vi "AlliGator Computer User-defined Quantity.vi"(6 "Init (F)":bool, 8 "Error In":errorcluster, 9 "Formula":string, 11 "Basic Quantities":sgl[](array[numeric])) -> (0 "Error Out":errorcluster, 3 "User-defined Quantity":sgl)   [LabVIEW 2021, in "AlliGator Phasor Plot.lvlib"]
doc: "Computes a user-defined quantity based on the basic quantities:\n\nf_!, f_2, a_1, a_2\ntau_phi, tau_m,\n<tau>_i, <tau>_a,\ntau_1, tau_@,\nT_laser, T_sync,\nN_gates,\ndt (gate separation)\nCh_INT (intensity of the INT channel)\nCh_G2 (intensity of the INT channel)"
uses:
  AlliGator Phasor Plot.lvlib
  <vilib>/gmath/NI_Gmath.lvlib
panel:
  # "see the AlliGator License on the block diagram (Ctrl+E or Window:Show Block Diagram)"
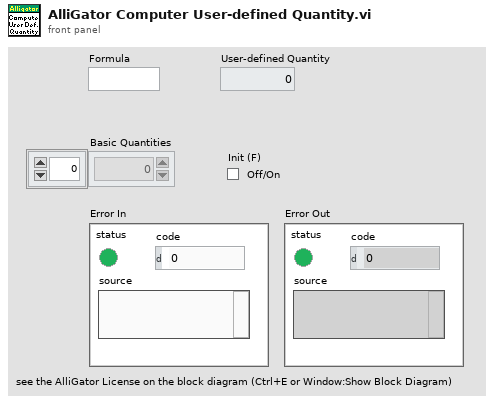
[diagram p1: front panel]
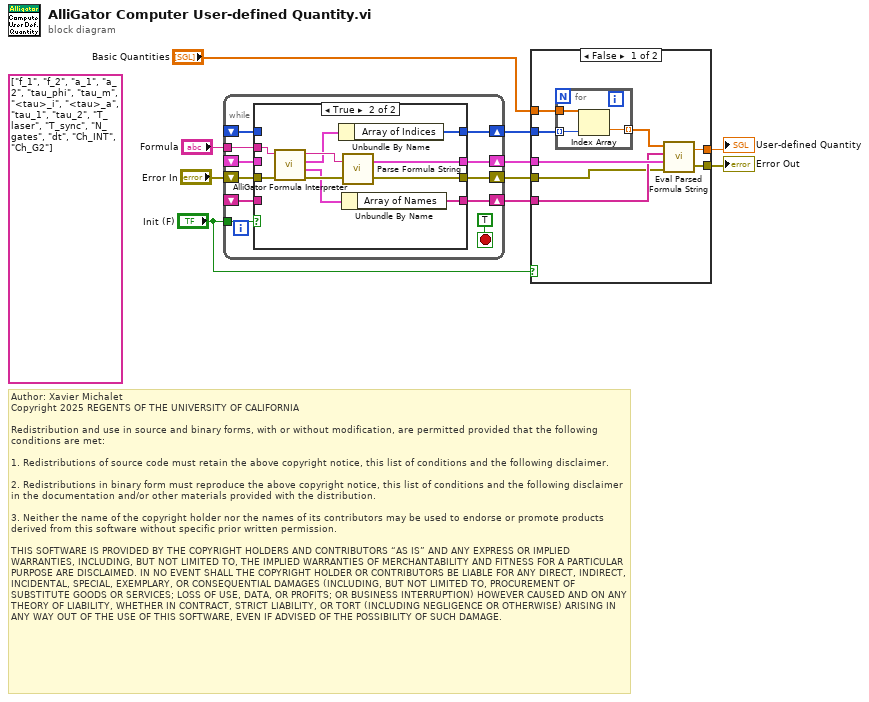
[diagram p0: block diagram]
diagram:
  (unwired) string[] ["f_1", "f_2", "a_1", "a_2", "tau_phi", "tau_m", "<tau>_i", "<tau>_a", "tau_1", "tau_2", "T_laser", "T_sync", "N_gates", "dt", "Ch_INT", "Ch_G2"] ("Basic Variable Names")
  # "Author: Xavier Michalet\nCopyright 2025 REGENTS OF THE UNIVERSITY OF CALIFORNIA\n\nRedistribution and use in source and binary forms, with or without modification, are permitted provided that the following conditions are met:\n\n1. Redistributions of source code must retain the above copyright notice, this list of conditions and the following disclaimer.\n\n2. Redistributions in binary form must reproduce the above copyright notice, this list of conditions and the following disclaimer in the documentation and/or other materials provided with the distribution.\n\n3. Neither the name of the copyright holder nor the names of its contributors may be used to endorse or promote products derived from this software without specific prior written permission.\n\nTHIS SOFTWARE IS PROVIDED BY THE COPYRIGHT HOLDERS AND CONTRIBUTORS “AS IS” AND ANY EXPRESS OR IMPLIED WARRANTIES, INCLUDING, BUT NOT LIMITED TO, THE IMPLIED WARRANTIES OF MERCHANTABILITY AND FITNESS FOR A PARTICULAR PURPOSE ARE DISCLAIMED. IN NO EVENT SHALL THE COPYRIGHT HOLDER OR CONTRIBUTORS BE LIABLE FOR ANY DIRECT, INDIRECT, INCIDENTAL, SPECIAL, EXEMPLARY, OR CONSEQUENTIAL DAMAGES (INCLUDING, BUT NOT LIMITED TO, PROCUREMENT OF SUBSTITUTE GOODS OR SERVICES; LOSS OF USE, DATA, OR PROFITS; OR BUSINESS INTERRUPTION) HOWEVER CAUSED AND ON ANY THEORY OF LIABILITY, WHETHER IN CONTRACT, STRICT LIABILITY, OR TORT (INCLUDING NEGLIGENCE OR OTHERWISE) ARISING IN ANY WAY OUT OF THE USE OF THIS SOFTWARE, EVEN IF ADVISED OF THE POSSIBILITY OF SUCH DAMAGE."
  n1 = while {
    tunnel: "Formula" -> [w21]
    shift-right: [w16] -> w4
    shift-left: "Error In" -> [w20]
    tunnel: "Init (F)" -> [w14]
    shift-right: [w19] -> w8
    shift-left: _ -> [w13]
    shift-right: [w18] -> w6
    shift-left: _ -> [w12]
    shift-right: [w17] -> w5
    shift-left: _ -> [w11]
    stop <- TRUE stop-if-true
    n2 = case shown="True" w14 {
      tunnel: w21 -> [_ w35]
      tunnel: w20 -> [w22 w34]
      tunnel: [w25 w30] -> w19
      tunnel: [w24 w29] -> w18
      tunnel: [w23 w27] -> w17
      tunnel: [w22 w26] -> w16
      tunnel: w13 -> [w25 _]
      tunnel: w12 -> [w24 _]
      tunnel: w11 -> [w23 _]
      frame False {
      }
      frame True {
        n3 = call "AlliGator Formula Interpreter.vi"("error in (no error)"=w34, "Original Formula"=w35) -> ("error out"=w32:errorcluster, "Variable Names"=w28:cluster{"Array of Names":string[]}, "Variable Indices"=w31:cluster{"Array of Indices":i32[]}, "Interpreted Formula"=w33:string)  [unwired: 5 in, 1 out]
        n4 = Unbundle By Name(w31) -> ("Array of Indices"=w30:i32[])
        n5 = Unbundle By Name(w28) -> ("Array of Names"=w27:string[])
        n6 = call <vilib>:"Parse Formula String.vi"("error in (no error)"=w32, "formula"=w33) -> ("error out"=w26:errorcluster, "Parsed Formula"=w29:cluster{"Table":i32[][], "Y Values":dbl[]})
      }
    }
  }
  n7 = case shown="False" "Init (F)" {
    tunnel: w8 -> [w42 _]
    tunnel: "Basic Quantities" -> [w41 _]
    tunnel: w6 -> [w40 _]
    tunnel: w5 -> [w39 _]
    tunnel: w4 -> [w38 w47]
    tunnel: [w37 w47] -> w3
    tunnel: [w36 _] -> w2
    frame False {
      n8 = for {
        tunnel: w42 -> [w44] mode=indexing
        tunnel: w41 -> [w46]
        tunnel: [w45] -> w43 mode=indexing
        n9 = Index Array(array=w46, index=w44) -> (element=w45:sgl)
      }
      n10 = call <vilib>:"Eval Parsed Formula String.vi"("error in (no error)"=w38, "Parsed Formula"=w40, "Variables"=w39, "X Values"=w43) -> ("error out"=w37:errorcluster, "y value"=w36:dbl)
    }
    frame True {
    }
  }
  "User-defined Quantity" <- w2
  "Error Out" <- w3
